vi "configuration_read.vi"(8 "error in (no error)":errorcluster, 11 "lv-build in":refnum<class "lv-builder.lvclass">) -> (0 "error out":errorcluster, 2 "configuration":variant, 3 "lv-build out":refnum<class "lv-builder.lvclass">)   [LabVIEW 2015, in "lv-builder.lvclass"]
uses:
  lv-builder.lvclass
  lv-builder.lvclass/lv-builder.ctl
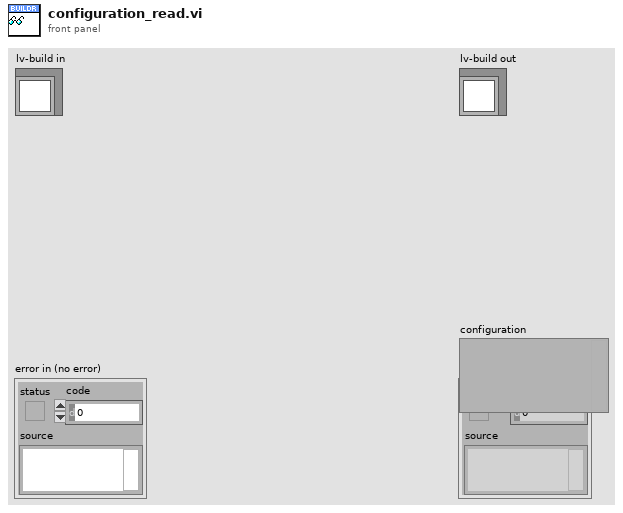
[diagram p1: front panel]
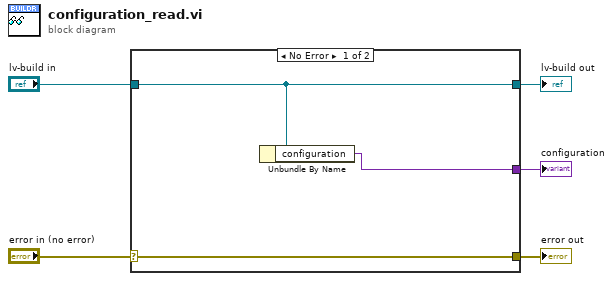
[diagram p0: block diagram]
diagram:
  n1 = case shown="No Error" "error in (no error)" {
    selector: "error in (no error)" -> [w8 w9]
    tunnel: [w8 w9] -> w4
    tunnel: [w7 w10] -> w2
    tunnel: "lv-build in" -> [w7 w10]
    tunnel: [w6 _] -> w1
    frame No Error {
      n2 = Unbundle By Name(w7) -> ("configuration"=w6:variant)
    }
    frame Error {
    }
  }
  "error out" <- w4
  "lv-build out" <- w2
  "configuration" <- w1
